vi "Auto Number Update.vi"(8 "error in (no error)":errorcluster, 10 "Auto Number Record":T2, 11 "Connection Refnum":T1) -> (0 "error out":errorcluster, 3 "Connection Refnum":T1)   [LabVIEW 2011]
uses:
  Auto Number Record.ctl
  SI.LIB/ODBC/SQL Controls/Connection Refnum.ctl
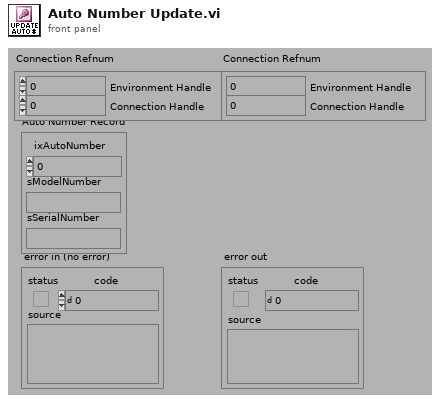
[diagram p1: front panel]
types:
  T1 = typedef "Connection Refnum.ctl" = cluster{"Environment Handle":i32, "Connection Handle":i32}
  T2 = typedef "Auto Number Record.ctl" = cluster{"ixAutoNumber":i32, "sModelNumber":string, "sSerialNumber":string}
  T3 = typedef "Statement Refnum.ctl" = cluster{"Statement Handle":i32, "Parameter Number":u16}
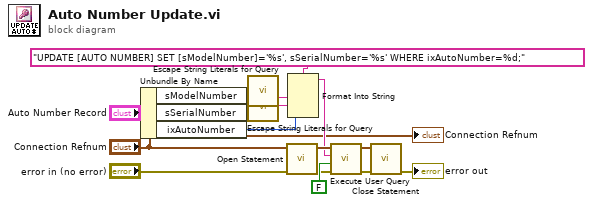
[diagram p0: block diagram]
diagram:
  n1 = Unbundle By Name("Auto Number Record") -> ("sModelNumber"=w6:string, "sSerialNumber"=w4:string, "ixAutoNumber"=w7:i32)
  n2 = call "Escape String Literals for Query.vi"("String"=w6) -> ("escaped String"=w5:string)  [unwired: 1 in, 13 out]
  n3 = call "Escape String Literals for Query.vi"("String"=w4) -> ("escaped String"=w3:string)  [unwired: 1 in, 13 out]
  n4 = call "Open Statement.vi"("error in (no error)"="error in (no error)", "Connection Refnum"="Connection Refnum") -> ("error out"=w13:errorcluster, "Statement Refnum"=w12:T3)  [unwired: 4 out]
  n5 = Format Into String(format string="UPDATE [AUTO NUMBER] SET [sModelNumber]='%s', sSerialNumber='%s' WHERE ixAutoNumber=%d;", w5, w3, w7) -> (resulting string=w10:string)  [unwired: 2 in, 1 out]
  n6 = call "Execute User Query.vi"("error in (no error)"=w13, "Return Data? (f)"=FALSE, "User Query"=w10, "Statement Refnum"=w12) -> ("error out"=w14:errorcluster, "Statement Refnum"=w15:T3)  [unwired: 2 out]
  n7 = call "Close Statement.vi"("error in (no error)"=w14, "Statement Refnum"=w15) -> ("error out"=→"error out":errorcluster)  [unwired: 5 out]
  "Connection Refnum" <- "Connection Refnum"
